vi "retrieveTable--string.vi"(8 "error in (no error)":errorcluster, 11 "MS-Excel in":refnum<class "MS-Excel.lvclass">) -> (0 "error out":errorcluster, 2 "Table":string[][](array[string]), 3 "MS-Excel out":refnum<class "MS-Excel.lvclass">)   [LabVIEW 2020, in "LabVIEW NPOI.lvlib" / "MS-Excel.lvclass"]
doc: "Protected dynamic dispatch method to append the wire <b>Table</b> as 2D array of strings to the <b>Document</b> as a table."
uses:
  MS-Excel.lvclass
  D:/Benjamin/Documents/Perso/Code/WC/LVExcel/Resources/NPOI 2.1.1 dotnet2/NPOI.dll
  LVExcel/Resources/NPOI 2.1.1 dotnet2/NPOI.dll
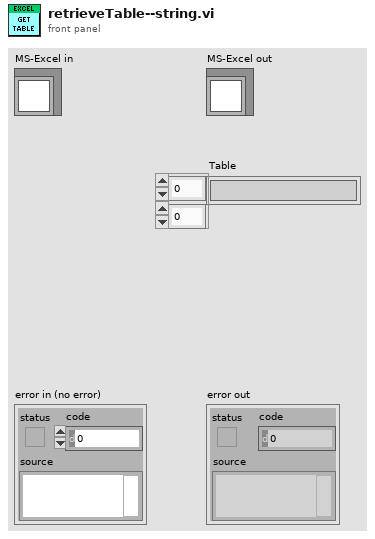
[diagram p1: front panel]
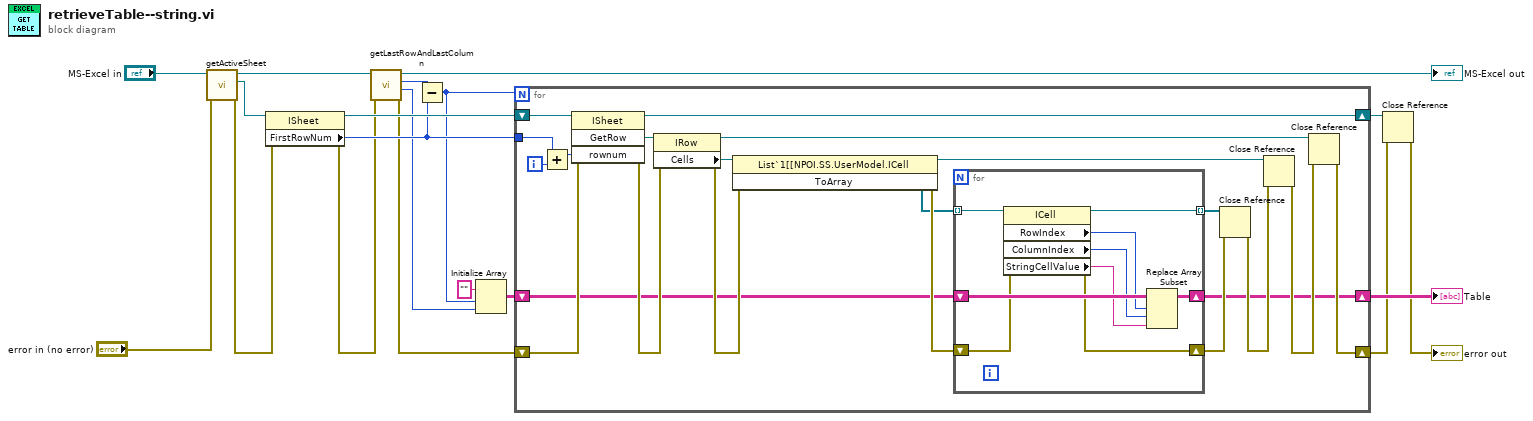
[diagram p0: block diagram]
diagram:
  n1 = call-dynamic "getActiveSheet.vi"("error in (no error)"="error in (no error)", "MS-Excel in"="MS-Excel in") -> ("error out"=w15:errorcluster, "Sheet Ref"=w17:refnum<k24>, "MS-Excel out"=w18:refnum<class "MS-Excel.lvclass">)  [unwired: 6 in, 1 out]
  n2 = property class="ISheet"(reference=w17, error in=w15) -> (reference out=w16:refnum<k24>, error out=w5:errorcluster, "FirstRowNum"=w13:i32)
  n3 = call-dynamic "getLastRowAndLastColumn.vi"("error in (no error)"=w5, "MS-Excel in"=w18) -> ("error out"=w4:errorcluster, "Last Column"=w7:i32, "Last Row"=w11:i32, "MS-Excel out"=→"MS-Excel out":refnum<class "MS-Excel.lvclass">)  [unwired: 6 in]
  n4 = Subtract(x=w11, y=w13) -> (x-y=w8:i32)
  n5 = Initialize Array("", w8, w7) -> (w6:string[][])
  n6 = for {
    N: w8 -> [_]
    shift-right: [w28] -> w2
    shift-left: w4 -> [w35]
    tunnel: w13 -> [w32]
    shift-right: [w29] -> w3
    shift-left: w16 -> [w40]
    shift-right: [w20] -> w10
    shift-left: w6 -> [w21]
    i -> [w30]
    n7 = Add(x=w32, y=w30) -> (x+y=w31:i32)
    n8 = invoke class="ISheet" method="GetRow"(reference=w40, error in=w35, "rownum"=w31) -> (reference out=w29:refnum<k24>, error out=w34:errorcluster, "GetRow"=w39:refnum<k24>)  [unwired: 1 in, 1 out]
    n9 = property class="IRow"(reference=w39, error in=w34) -> (reference out=w36:refnum<k24>, error out=w33:errorcluster, "Cells"=w27:refnum<k24>)
    n10 = invoke class="List`1[[NPOI.SS.UserModel.ICell" method="ToArray"(reference=w27, error in=w33) -> (reference out=w38:refnum<k24>, error out=w26:errorcluster, "ToArray"=w25:refnum<k24>[])  [unwired: 1 in]
    n11 = for {
      tunnel: w25 -> [w49] mode=indexing
      shift-right: [w42] -> w23
      shift-left: w26 -> [w44]
      tunnel: [w43] -> w24 mode=indexing
      shift-right: [w47] -> w20
      shift-left: w21 -> [w48]
      n12 = property class="ICell"(reference=w49, error in=w44) -> (reference out=w43:refnum<k24>, error out=w42:errorcluster, "RowIndex"=w46:i32, "ColumnIndex"=w45:i32, "StringCellValue"=w41:string)
      n13 = Replace Array Subset(array=w48, new element=w41, index (row)=w46, index (col)=w45) -> (w47:string[][])
    }
    n14 = Close Reference(reference=w24, error in (no error)=w23) -> (error out=w22:errorcluster)
    n15 = Close Reference(reference=w38, error in (no error)=w22) -> (error out=w37:errorcluster)
    n16 = Close Reference(reference=w36, error in (no error)=w37) -> (error out=w28:errorcluster)
  }
  "Table" <- w10
  n17 = Close Reference(reference=w3, error in (no error)=w2) -> (error out=→"error out":errorcluster)
